vi "set_register_bits.vi"(11 "Array in":bool[](array[boolean])) -> (3 "Array out":u8[](array[numeric]))   [LabVIEW 2021]
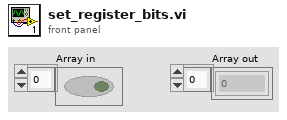
[diagram p1: front panel]
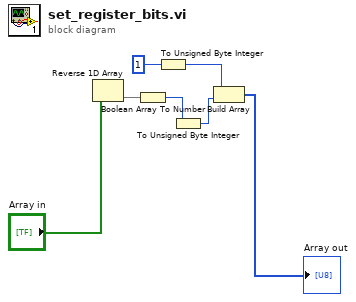
[diagram p0: block diagram]
diagram:
  n1 = Reverse 1D Array(array="Array in") -> (reversed array=w2:bool[])
  n2 = Boolean Array To Number(Boolean array=w2) -> (number=w3:u32)
  n3 = To Unsigned Byte Integer(number=u8 1) -> (unsigned 8bit integer=w6:u8)
  n4 = To Unsigned Byte Integer(number=w3) -> (unsigned 8bit integer=w5:u8)
  n5 = Build Array(w6, w5) -> (→"Array out":u8[])
